vi "charts_yscale_temperature.vi"(8 "error in":errorcluster, 9 "padding":sgl=0.1, 10 "vars general":T1[](array[typedef]) {"stim ramp" min=1}, 11 "control cluster":T4) -> (0 "error out":errorcluster, 2 "vars general":T1[](array[typedef]) {"stim ramp" min=1}, 3 "control cluster":T4)   [LabVIEW 2016]
uses:
  Type Definitions/control_references.ctl
  Type Definitions/vars_settings.ctl
  Type Definitions/stim_type.ctl
  Type Definitions/backlight_type.ctl
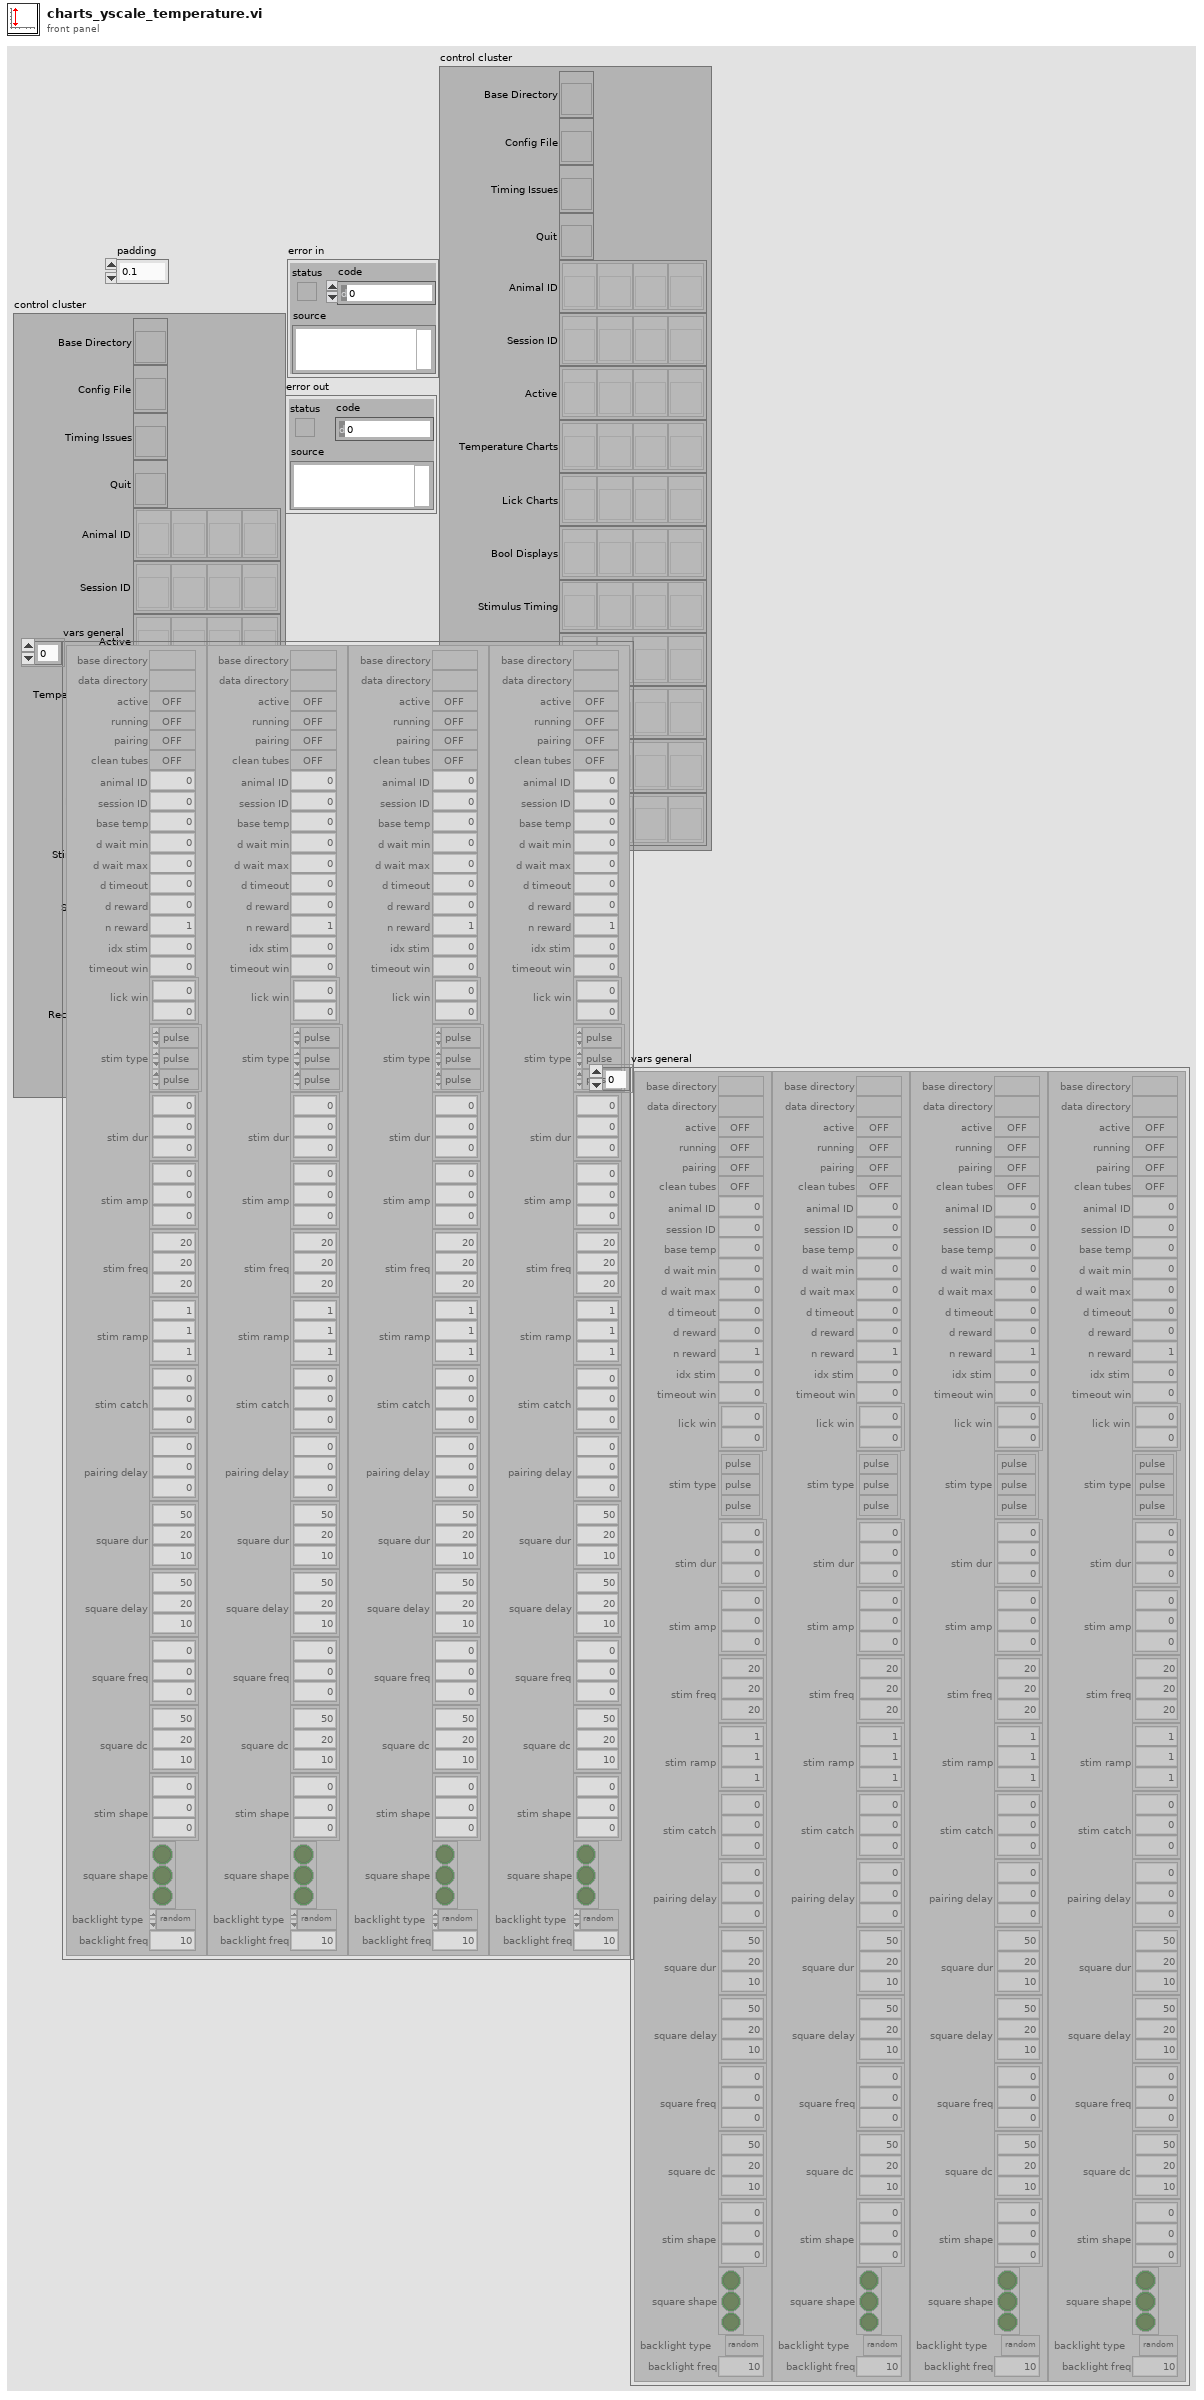
[diagram p1: front panel]
types:
  T1 = typedef "vars_settings.ctl" = cluster{"base directory":path, "data directory":path, "active":bool, "running":bool, "pairing":bool, "clean tubes":bool, "animal ID":u16, "session ID":u16, "base temp":dbl, "d wait min":u16, "d wait max":u16, "d timeout":u16, "d reward":u16, "n reward":u16, "idx stim":u16, "timeout win":u16, "lick win":i32[], "stim type":T2[], "stim dur":u16[], "stim amp":dbl[], "stim freq":u16[], "stim ramp":u16[], "stim catch":u8[], "pairing delay":i16[], "square dur":u16[], "square delay":i16[], "square freq":u8[], "square dc":u8[], "stim shape":dbl[][], "square shape":bool[][], "backlight type":T3, "backlight freq":u16}
  T2 = typedef "stim_type.ctl" = enum16{"pulse", "vibration", "square", "sine"}
  T3 = typedef "backlight_type.ctl" = enum16{"none", "random", "regular"}
  T4 = typedef "control_references.ctl" = cluster{"Base Directory":refnum<vi>, "Config File":refnum<vi>, "Timing Issues":refnum<vi>, "Quit":refnum<vi>, "Animal ID":refnum<vi>[], "Session ID":refnum<vi>[], "Active":refnum<vi>[], "Temperature Charts":refnum<vi>[], "Lick Charts":refnum<vi>[], "Bool Displays":refnum<vi>[], "Stimulus Timing":refnum<vi>[], "Stimulus Stats":refnum<vi>[], "Catch Stats":refnum<vi>[], "Recording Status":refnum<vi>[], "Pairing":refnum<vi>[]}
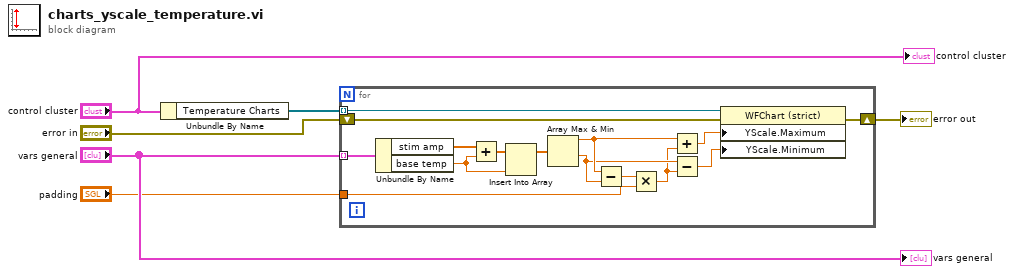
[diagram p0: block diagram]
diagram:
  n1 = Unbundle By Name("control cluster") -> ("Temperature Charts"=w5:refnum<vi>[])
  n2 = for {
    tunnel: w5 -> [w21] mode=indexing
    tunnel: "vars general" -> [w20] mode=indexing
    shift-right: [w9] -> w4
    shift-left: "error in" -> [w8]
    tunnel: "padding" -> [w7]
    n3 = Unbundle By Name(w20) -> ("stim amp"=w19:dbl[], "base temp"=w17:dbl)
    n4 = Add(x=w19, y=w17) -> (x+y=w18:dbl[])
    n5 = Insert Into Array(array=w18, new element=w17) -> (w16:dbl[])  [unwired: 1 in]
    n6 = Array Max & Min(array=w16) -> (max value=w14:dbl, min value=w13:dbl)  [unwired: 2 out]
    n7 = Subtract(x=w14, y=w13) -> (x-y=w15:dbl)
    n8 = Multiply(x=w15, y=w7) -> (x*y=w12:dbl)
    n9 = Add(x=w14, y=w12) -> (x+y=w11:dbl)
    n10 = Subtract(x=w13, y=w12) -> (x-y=w10:dbl)
    n11 = property class="WFChart (strict)"(reference=w21, error in=w8, "YScale.Maximum"=w11, "YScale.Minimum"=w10) -> (error out=w9:errorcluster)  [unwired: 1 out]
  }
  "error out" <- w4
  "control cluster" <- "control cluster"
  "vars general" <- "vars general"
